vi "Goo00.vi"() -> ()   [LabVIEW 2014]
uses:
  <vilib>/myRIO/Instrument Drivers/Onboard IO/AI/vis/Read.vi
  <vilib>/myRIO/Instrument Drivers/Onboard IO/AI/vis/Smart Open.vi
  <vilib>/Utility/error.llb/Error Cluster From Error Code.vi
  <vilib>/myRIO/Common/Instrument Driver Framework/myRIO v1.0/AI/vis/myRIO v1.0 Read AI.vi
panel:
  out "원소의 인덱스":i32
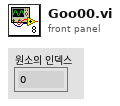
[diagram p1: front panel]
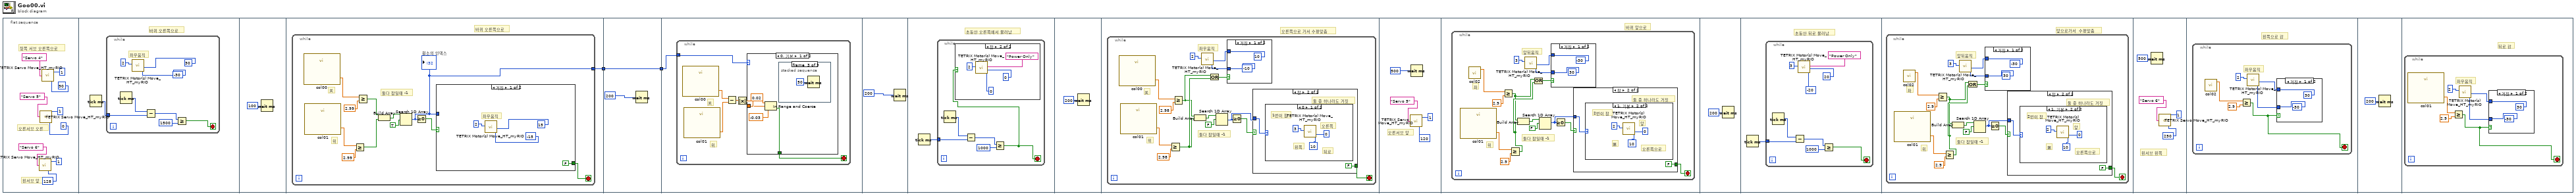
[diagram p0: block diagram]
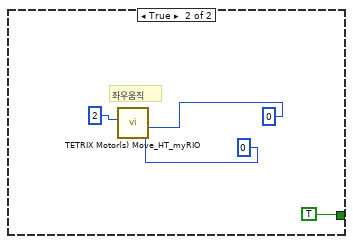
[diagram p2: hidden frame]
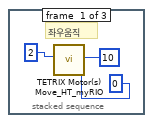
[diagram p3: hidden frame]
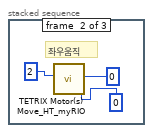
[diagram p4: hidden frame]
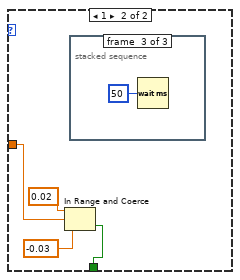
[diagram p5: hidden frame]
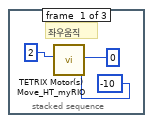
[diagram p6: hidden frame]
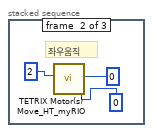
[diagram p7: hidden frame]
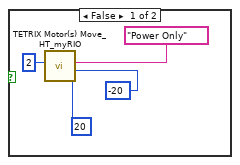
[diagram p8: hidden frame]
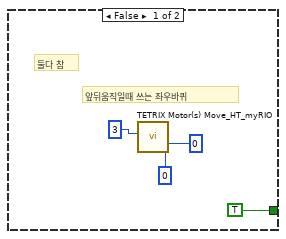
[diagram p9: hidden frame]
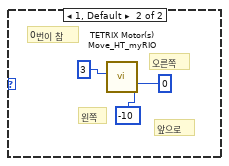
[diagram p10: hidden frame]
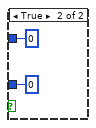
[diagram p11: hidden frame]
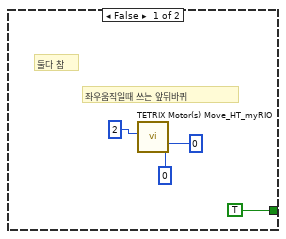
[diagram p12: hidden frame]
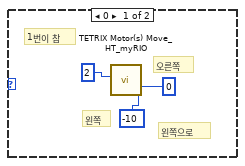
[diagram p13: hidden frame]
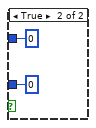
[diagram p14: hidden frame]
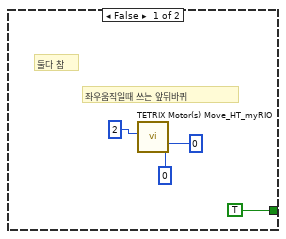
[diagram p15: hidden frame]
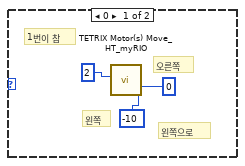
[diagram p16: hidden frame]
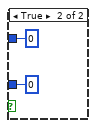
[diagram p17: hidden frame]
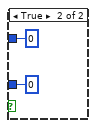
[diagram p18: hidden frame]
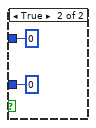
[diagram p19: hidden frame]
diagram:
  n1 = flat-sequence {
    tunnel: [w22] -> w1
    tunnel: [w42] -> w2
    tunnel: w1 -> [w42]
    tunnel: w2 -> [w44]
    frame #0 {
      # "왼서브 앞"
      # "오른서브 오른"
      # "뒷쪽 서브 오른쪽으로"
      n2 = call <vilib>:"TETRIX Servo Move_HT_myRIO.vi"("Servo Position (0 - 255)"=u8 128, "Controller Daisy Chain Position (1 - 4)"=u8 1, "Select Servo"="Servo 6") -> ()  [unwired: 2 in, 1 out]
      n3 = call <vilib>:"TETRIX Servo Move_HT_myRIO.vi"("Servo Position (0 - 255)"=u8 0, "Controller Daisy Chain Position (1 - 4)"=u8 1, "Select Servo"="Servo 5") -> ()  [unwired: 2 in, 1 out]
      n4 = call <vilib>:"TETRIX Servo Move_HT_myRIO.vi"("Servo Position (0 - 255)"=u8 90, "Controller Daisy Chain Position (1 - 4)"=u8 1, "Select Servo"="Servo 4") -> ()  [unwired: 2 in, 1 out]
    }
    frame #1 {
      # "바퀴 오른쪽으로"
      n5 = Tick Count (ms)() -> (millisecond timer value=w12:u32)
      n6 = while {
        tunnel: w12 -> [w16]
        stop <- w13 stop-if-true
        # "좌우움직"
        n7 = Tick Count (ms)() -> (millisecond timer value=w17:u32)
        n8 = call <vilib>:"TETRIX Motor(s) Move_HT_myRIO.vi"("Motor 2 Power (-100 to 100)\n0 = Stop/Brake\n-128 = Stop/Coast"=i8 -30 ("Motor 2 Power (-100 to 100)\n0 = Stop/Brake\n-128 = Stop/Coast"), "Motor 1 Power (-100 to 100)\n0 = Stop/Brake\n-128 = Stop/Coast"=i8 30 ("Motor 1 Power (-100 to 100)\n0 = Stop/Brake\n-128 = Stop/Coast"), "Controller Daisy Chain Position: 1 - 4"=u8 2) -> ()  [unwired: 6 in, 1 out]
        n9 = Subtract(x=w17, y=w16) -> (x-y=w15:u32)
        n10 = Greater Or Equal?(x=w15, y=u32 1500) -> (x >= y?=w13:bool)
      }
    }
    frame #2 {
      n11 = Wait (ms)(milliseconds to wait=u32 100 ("대기 시간(ms)")) -> ()  [unwired: 1 out]
    }
    frame #3 {
      # "바퀴 오른쪽으로"
      n12 = while {
        tunnel: [w23] -> w22
        stop <- w26 stop-if-true
        # "위"
        # "关"
        # "둘다 참일때 -1"
        n13 = call "col00.vi"() -> ("Col00 (B/AI0 (Pin 3))"=w25:dbl)  [unwired: 26 in, 1 out]
        n14 = call "col01.vi"() -> ("Col01 (B/AI1 (Pin 5))"=w24:dbl)  [unwired: 26 in, 1 out]
        n15 = Greater Or Equal?(x=w24, y=2.99) -> (x >= y?=w30:bool)
        n16 = Greater Or Equal?(x=w25, y=2.99) -> (x >= y?=w29:bool)
        n17 = Build Array(w29, w30) -> (w33:bool[])
        n18 = Search 1D Array(1D array=w33, element=TRUE ("원소")) -> (index of element=w23:i32)  [unwired: 1 in]
        "원소의 인덱스" <- w23
        n19 = Greater Or Equal To 0?(x=w23) -> (x >= 0?=w31:bool)
        n20 = case shown="거짓" w31 {
          tunnel: w23 -> [_ _]
          tunnel: [FALSE TRUE] -> w26
          frame False {
            # "좌우움직"
            n21 = call <vilib>:"TETRIX Motor(s) Move_HT_myRIO.vi"("Motor 2 Power (-100 to 100)\n0 = Stop/Brake\n-128 = Stop/Coast"=i8 -15 ("Motor 2 Power (-100 to 100)\n0 = Stop/Brake\n-128 = Stop/Coast"), "Motor 1 Power (-100 to 100)\n0 = Stop/Brake\n-128 = Stop/Coast"=i8 15 ("Motor 1 Power (-100 to 100)\n0 = Stop/Brake\n-128 = Stop/Coast"), "Controller Daisy Chain Position: 1 - 4"=u8 2) -> ()  [unwired: 6 in, 1 out]
          }
          frame True {
            # "좌우움직"
            n22 = call <vilib>:"TETRIX Motor(s) Move_HT_myRIO.vi"("Motor 2 Power (-100 to 100)\n0 = Stop/Brake\n-128 = Stop/Coast"=i8 0 ("Motor 2 Power (-100 to 100)\n0 = Stop/Brake\n-128 = Stop/Coast"), "Motor 1 Power (-100 to 100)\n0 = Stop/Brake\n-128 = Stop/Coast"=i8 0 ("Motor 1 Power (-100 to 100)\n0 = Stop/Brake\n-128 = Stop/Coast"), "Controller Daisy Chain Position: 1 - 4"=u8 2) -> ()  [unwired: 6 in, 1 out]
          }
        }
      }
    }
    frame #4 {
      n23 = Wait (ms)(milliseconds to wait=u32 200 ("대기 시간(ms)")) -> ()  [unwired: 1 out]
    }
    frame #5 {
      n24 = while {
        tunnel: w44 -> [w50]
        stop <- w45 stop-if-true
        # "위"
        # "关"
        n25 = call "col00.vi"() -> ("Col00 (B/AI0 (Pin 3))"=w49:dbl)  [unwired: 26 in, 1 out]
        n26 = call "col01.vi"() -> ("Col01 (B/AI1 (Pin 5))"=w48:dbl)  [unwired: 26 in, 1 out]
        n27 = Subtract(x=w49, y=w48) -> (x-y=w47:dbl)
        n28 = Absolute Value(x=w47) -> (abs(x)=w46:dbl)
        n29 = case shown="0, 기본" w50 {
          tunnel: w46 -> [w54 w63]
          tunnel: [w51 w62] -> w45
          frame 0, Default {
            n30 = In Range and Coerce(upper limit=0.02 ("상위 리미트"), x=w54, lower limit=-0.03 ("상위 리미트")) -> (In Range?=w51:bool)  [unwired: 1 out]
            n31 = stacked-sequence {
              frame #0 {
                # "좌우움직"
                n32 = call <vilib>:"TETRIX Motor(s) Move_HT_myRIO.vi"("Motor 2 Power (-100 to 100)\n0 = Stop/Brake\n-128 = Stop/Coast"=i8 0 ("Motor 2 Power (-100 to 100)\n0 = Stop/Brake\n-128 = Stop/Coast"), "Motor 1 Power (-100 to 100)\n0 = Stop/Brake\n-128 = Stop/Coast"=i8 10 ("Motor 1 Power (-100 to 100)\n0 = Stop/Brake\n-128 = Stop/Coast"), "Controller Daisy Chain Position: 1 - 4"=u8 2) -> ()  [unwired: 6 in, 1 out]
              }
              frame #1 {
                # "좌우움직"
                n33 = call <vilib>:"TETRIX Motor(s) Move_HT_myRIO.vi"("Motor 2 Power (-100 to 100)\n0 = Stop/Brake\n-128 = Stop/Coast"=i8 0 ("Motor 2 Power (-100 to 100)\n0 = Stop/Brake\n-128 = Stop/Coast"), "Motor 1 Power (-100 to 100)\n0 = Stop/Brake\n-128 = Stop/Coast"=i8 0 ("Motor 1 Power (-100 to 100)\n0 = Stop/Brake\n-128 = Stop/Coast"), "Controller Daisy Chain Position: 1 - 4"=u8 2) -> ()  [unwired: 6 in, 1 out]
              }
              frame #2 {
                n34 = Wait (ms)(milliseconds to wait=u32 50 ("대기 시간(ms)")) -> ()  [unwired: 1 out]
              }
            }
          }
          frame 1 {
            n35 = In Range and Coerce(upper limit=0.02 ("상위 리미트"), x=w63, lower limit=-0.03 ("상위 리미트")) -> (In Range?=w62:bool)  [unwired: 1 out]
            n36 = stacked-sequence {
              frame #0 {
                # "좌우움직"
                n37 = call <vilib>:"TETRIX Motor(s) Move_HT_myRIO.vi"("Motor 2 Power (-100 to 100)\n0 = Stop/Brake\n-128 = Stop/Coast"=i8 -10 ("Motor 2 Power (-100 to 100)\n0 = Stop/Brake\n-128 = Stop/Coast"), "Motor 1 Power (-100 to 100)\n0 = Stop/Brake\n-128 = Stop/Coast"=i8 0 ("Motor 1 Power (-100 to 100)\n0 = Stop/Brake\n-128 = Stop/Coast"), "Controller Daisy Chain Position: 1 - 4"=u8 2) -> ()  [unwired: 6 in, 1 out]
              }
              frame #1 {
                # "좌우움직"
                n38 = call <vilib>:"TETRIX Motor(s) Move_HT_myRIO.vi"("Motor 2 Power (-100 to 100)\n0 = Stop/Brake\n-128 = Stop/Coast"=i8 0 ("Motor 2 Power (-100 to 100)\n0 = Stop/Brake\n-128 = Stop/Coast"), "Motor 1 Power (-100 to 100)\n0 = Stop/Brake\n-128 = Stop/Coast"=i8 0 ("Motor 1 Power (-100 to 100)\n0 = Stop/Brake\n-128 = Stop/Coast"), "Controller Daisy Chain Position: 1 - 4"=u8 2) -> ()  [unwired: 6 in, 1 out]
              }
              frame #2 {
                n39 = Wait (ms)(milliseconds to wait=u32 50 ("대기 시간(ms)")) -> ()  [unwired: 1 out]
              }
            }
          }
        }
      }
    }
    frame #6 {
      n40 = Wait (ms)(milliseconds to wait=u32 200 ("대기 시간(ms)")) -> ()  [unwired: 1 out]
    }
    frame #7 {
      # "초동안 오른쪽에서 물러남"
      n41 = Tick Count (ms)() -> (millisecond timer value=w74:u32)
      n42 = while {
        tunnel: w74 -> [w78]
        stop <- w75 stop-if-true
        n43 = Tick Count (ms)() -> (millisecond timer value=w79:u32)
        n44 = Subtract(x=w79, y=w78) -> (x-y=w77:u32)
        n45 = Greater Or Equal?(x=w77, y=u32 1000) -> (x >= y?=w75:bool)
        n46 = case shown="참" w75 {
          frame False {
            n47 = call <vilib>:"TETRIX Motor(s) Move_HT_myRIO.vi"("Motor 2 Power (-100 to 100)\n0 = Stop/Brake\n-128 = Stop/Coast"=i8 20 ("Motor 2 Power (-100 to 100)\n0 = Stop/Brake\n-128 = Stop/Coast"), "Motor 1 Power (-100 to 100)\n0 = Stop/Brake\n-128 = Stop/Coast"=i8 -20 ("Motor 1 Power (-100 to 100)\n0 = Stop/Brake\n-128 = Stop/Coast"), "Control Mode"="Power Only", "Controller Daisy Chain Position: 1 - 4"=u8 2) -> ()  [unwired: 5 in, 1 out]
          }
          frame True {
            n48 = call <vilib>:"TETRIX Motor(s) Move_HT_myRIO.vi"("Motor 2 Power (-100 to 100)\n0 = Stop/Brake\n-128 = Stop/Coast"=i8 0 ("Motor 2 Power (-100 to 100)\n0 = Stop/Brake\n-128 = Stop/Coast"), "Motor 1 Power (-100 to 100)\n0 = Stop/Brake\n-128 = Stop/Coast"=i8 0 ("Motor 1 Power (-100 to 100)\n0 = Stop/Brake\n-128 = Stop/Coast"), "Control Mode"="Power Only", "Controller Daisy Chain Position: 1 - 4"=u8 2) -> ()  [unwired: 5 in, 1 out]
          }
        }
      }
    }
    frame #8 {
      n49 = Wait (ms)(milliseconds to wait=u32 200 ("대기 시간(ms)")) -> ()  [unwired: 1 out]
    }
    frame #9 {
      # "오른쪽으로 가서 수평맞춤"
      n50 = while {
        stop <- w93 stop-if-true
        # "위"
        # "关"
        # "둘다 참일때 -1"
        # "좌우움직"
        n51 = call "col00.vi"() -> ("Col00 (B/AI0 (Pin 3))"=w91:dbl)  [unwired: 26 in, 1 out]
        n52 = call "col01.vi"() -> ("Col01 (B/AI1 (Pin 5))"=w92:dbl)  [unwired: 26 in, 1 out]
        n53 = Greater Or Equal?(x=w92, y=2.98) -> (x >= y?=w95:bool)
        n54 = Greater Or Equal?(x=w91, y=2.98) -> (x >= y?=w94:bool)
        n55 = Build Array(w94, w95) -> (w100:bool[])
        n56 = Or(x=w94, y=w95) -> (x .or. y?=w96:bool)
        n57 = Search 1D Array(1D array=w100, element=FALSE ("원소")) -> (index of element=w97:i32)  [unwired: 1 in]
        n58 = case shown="거짓" w96 {
          tunnel: [i8 10 ("Motor 1 Power (-100 to 100)\n0 = Stop/Brake\n-128 = Stop/Coast") i8 0 ("Motor 1 Power (-100 to 100)\n0 = Stop/Brake\n-128 = Stop/Coast")] -> w102
          tunnel: [i8 -10 ("Motor 2 Power (-100 to 100)\n0 = Stop/Brake\n-128 = Stop/Coast") i8 0 ("Motor 2 Power (-100 to 100)\n0 = Stop/Brake\n-128 = Stop/Coast")] -> w101
          frame False {
          }
          frame True {
          }
        }
        n59 = call <vilib>:"TETRIX Motor(s) Move_HT_myRIO.vi"("Motor 2 Power (-100 to 100)\n0 = Stop/Brake\n-128 = Stop/Coast"=w101, "Motor 1 Power (-100 to 100)\n0 = Stop/Brake\n-128 = Stop/Coast"=w102, "Controller Daisy Chain Position: 1 - 4"=u8 2) -> ()  [unwired: 6 in, 1 out]
        n60 = Greater Or Equal To 0?(x=w97) -> (x >= 0?=w98:bool)
        n61 = case shown="참" w98 {
          tunnel: w97 -> [_ w109]
          tunnel: [TRUE FALSE] -> w93
          frame False {
            # "앞뒤움직일때 쓰는 좌우바퀴"
            # "둘다 참"
            n62 = call <vilib>:"TETRIX Motor(s) Move_HT_myRIO.vi"("Motor 2 Power (-100 to 100)\n0 = Stop/Brake\n-128 = Stop/Coast"=i8 0 ("Motor 2 Power (-100 to 100)\n0 = Stop/Brake\n-128 = Stop/Coast"), "Motor 1 Power (-100 to 100)\n0 = Stop/Brake\n-128 = Stop/Coast"=i8 0 ("Motor 1 Power (-100 to 100)\n0 = Stop/Brake\n-128 = Stop/Coast"), "Controller Daisy Chain Position: 1 - 4"=u8 3) -> ()  [unwired: 6 in, 1 out]
          }
          frame True {
            # "둘 중 하나라도 거짓"
            n63 = case shown="0" w109 {
              frame 0 {
                # "뒤로"
                # "왼쪽"
                # "오른쪽"
                # "1번이 참"
                n64 = call <vilib>:"TETRIX Motor(s) Move_HT_myRIO.vi"("Motor 2 Power (-100 to 100)\n0 = Stop/Brake\n-128 = Stop/Coast"=i8 10 ("Motor 2 Power (-100 to 100)\n0 = Stop/Brake\n-128 = Stop/Coast"), "Motor 1 Power (-100 to 100)\n0 = Stop/Brake\n-128 = Stop/Coast"=i8 0 ("Motor 1 Power (-100 to 100)\n0 = Stop/Brake\n-128 = Stop/Coast"), "Controller Daisy Chain Position: 1 - 4"=u8 3) -> ()  [unwired: 6 in, 1 out]
              }
              frame 1, Default {
                # "앞으로"
                # "왼쪽"
                # "오른쪽"
                # "0번이 참"
                n65 = call <vilib>:"TETRIX Motor(s) Move_HT_myRIO.vi"("Motor 2 Power (-100 to 100)\n0 = Stop/Brake\n-128 = Stop/Coast"=i8 -10 ("Motor 2 Power (-100 to 100)\n0 = Stop/Brake\n-128 = Stop/Coast"), "Motor 1 Power (-100 to 100)\n0 = Stop/Brake\n-128 = Stop/Coast"=i8 0 ("Motor 1 Power (-100 to 100)\n0 = Stop/Brake\n-128 = Stop/Coast"), "Controller Daisy Chain Position: 1 - 4"=u8 3) -> ()  [unwired: 6 in, 1 out]
              }
            }
          }
        }
      }
    }
    frame #10 {
      # "오른서브 앞"
      n66 = call <vilib>:"TETRIX Servo Move_HT_myRIO.vi"("Servo Position (0 - 255)"=u8 120, "Controller Daisy Chain Position (1 - 4)"=u8 1, "Select Servo"="Servo 5") -> ()  [unwired: 2 in, 1 out]
      n67 = Wait (ms)(milliseconds to wait=u32 500 ("대기 시간(ms)")) -> ()  [unwired: 1 out]
    }
    frame #11 {
      # "바퀴 앞으로"
      n68 = while {
        stop <- w132 stop-if-true
        # "위"
        # "둘다 참일때 -1"
        # "앞뒤움직"
        # "좌"
        n69 = call "col01.vi"() -> ("Col01 (B/AI1 (Pin 5))"=w131:dbl)  [unwired: 26 in, 1 out]
        n70 = call "col02.vi"() -> ("Col02 (B/AI2 (Pin 7))"=w128:dbl)  [unwired: 26 in, 1 out]
        n71 = Greater Or Equal?(x=w128, y=2.9) -> (x >= y?=w124:bool)
        n72 = Greater Or Equal?(x=w131, y=2.9) -> (x >= y?=w125:bool)
        n73 = Build Array(w124, w125) -> (w127:bool[])
        n74 = Or(x=w124, y=w125) -> (x .or. y?=w133:bool)
        n75 = Search 1D Array(1D array=w127, element=FALSE ("원소")) -> (index of element=w134:i32)  [unwired: 1 in]
        n76 = case shown="거짓" w133 {
          tunnel: [i8 -30 ("Motor 1 Power (-100 to 100)\n0 = Stop/Brake\n-128 = Stop/Coast") i8 0 ("Motor 1 Power (-100 to 100)\n0 = Stop/Brake\n-128 = Stop/Coast")] -> w137
          tunnel: [i8 30 ("Motor 2 Power (-100 to 100)\n0 = Stop/Brake\n-128 = Stop/Coast") i8 0 ("Motor 2 Power (-100 to 100)\n0 = Stop/Brake\n-128 = Stop/Coast")] -> w136
          frame False {
          }
          frame True {
          }
        }
        n77 = call <vilib>:"TETRIX Motor(s) Move_HT_myRIO.vi"("Motor 2 Power (-100 to 100)\n0 = Stop/Brake\n-128 = Stop/Coast"=w136, "Motor 1 Power (-100 to 100)\n0 = Stop/Brake\n-128 = Stop/Coast"=w137, "Controller Daisy Chain Position: 1 - 4"=u8 3) -> ()  [unwired: 6 in, 1 out]
        n78 = Greater Or Equal To 0?(x=w134) -> (x >= 0?=w135:bool)
        n79 = case shown="참" w135 {
          tunnel: w134 -> [_ w144]
          tunnel: [TRUE FALSE] -> w132
          frame False {
            # "좌우움직일때 쓰는 앞뒤바퀴"
            # "둘다 참"
            n80 = call <vilib>:"TETRIX Motor(s) Move_HT_myRIO.vi"("Motor 2 Power (-100 to 100)\n0 = Stop/Brake\n-128 = Stop/Coast"=i8 0 ("Motor 2 Power (-100 to 100)\n0 = Stop/Brake\n-128 = Stop/Coast"), "Motor 1 Power (-100 to 100)\n0 = Stop/Brake\n-128 = Stop/Coast"=i8 0 ("Motor 1 Power (-100 to 100)\n0 = Stop/Brake\n-128 = Stop/Coast"), "Controller Daisy Chain Position: 1 - 4"=u8 2) -> ()  [unwired: 6 in, 1 out]
          }
          frame True {
            # "둘 중 하나라도 거짓"
            n81 = case shown="1, 기본" w144 {
              frame 0 {
                # "왼쪽으로"
                # "왼쪽"
                # "오른쪽"
                # "1번이 참"
                n82 = call <vilib>:"TETRIX Motor(s) Move_HT_myRIO.vi"("Motor 2 Power (-100 to 100)\n0 = Stop/Brake\n-128 = Stop/Coast"=i8 -10 ("Motor 2 Power (-100 to 100)\n0 = Stop/Brake\n-128 = Stop/Coast"), "Motor 1 Power (-100 to 100)\n0 = Stop/Brake\n-128 = Stop/Coast"=i8 0 ("Motor 1 Power (-100 to 100)\n0 = Stop/Brake\n-128 = Stop/Coast"), "Controller Daisy Chain Position: 1 - 4"=u8 2) -> ()  [unwired: 6 in, 1 out]
              }
              frame 1, Default {
                # "오른쪽으로"
                # "第"
                # "앞"
                # "2번이 참"
                n83 = call <vilib>:"TETRIX Motor(s) Move_HT_myRIO.vi"("Motor 2 Power (-100 to 100)\n0 = Stop/Brake\n-128 = Stop/Coast"=i8 10 ("Motor 2 Power (-100 to 100)\n0 = Stop/Brake\n-128 = Stop/Coast"), "Motor 1 Power (-100 to 100)\n0 = Stop/Brake\n-128 = Stop/Coast"=i8 0 ("Motor 1 Power (-100 to 100)\n0 = Stop/Brake\n-128 = Stop/Coast"), "Controller Daisy Chain Position: 1 - 4"=u8 2) -> ()  [unwired: 6 in, 1 out]
              }
            }
          }
        }
      }
    }
    frame #12 {
      n84 = Wait (ms)(milliseconds to wait=u32 200 ("대기 시간(ms)")) -> ()  [unwired: 1 out]
    }
    frame #13 {
      # "초동안 뒤로 물러남"
      n85 = Tick Count (ms)() -> (millisecond timer value=w156:u32)
      n86 = while {
        tunnel: w156 -> [w162]
        stop <- w159 stop-if-true
        n87 = Tick Count (ms)() -> (millisecond timer value=w163:u32)
        n88 = Subtract(x=w163, y=w162) -> (x-y=w161:u32)
        n89 = call <vilib>:"TETRIX Motor(s) Move_HT_myRIO.vi"("Motor 2 Power (-100 to 100)\n0 = Stop/Brake\n-128 = Stop/Coast"=i8 -20 ("Motor 2 Power (-100 to 100)\n0 = Stop/Brake\n-128 = Stop/Coast"), "Motor 1 Power (-100 to 100)\n0 = Stop/Brake\n-128 = Stop/Coast"=i8 20 ("Motor 1 Power (-100 to 100)\n0 = Stop/Brake\n-128 = Stop/Coast"), "Control Mode"="Power Only", "Controller Daisy Chain Position: 1 - 4"=u8 3) -> ()  [unwired: 5 in, 1 out]
        n90 = Greater Or Equal?(x=w161, y=u32 1000) -> (x >= y?=w159:bool)
      }
    }
    frame #14 {
      # "앞으로가서  수평맞춤"
      n91 = while {
        stop <- w174 stop-if-true
        # "위"
        # "둘다 참일때 -1"
        # "앞뒤움직"
        # "좌"
        n92 = call "col01.vi"() -> ("Col01 (B/AI1 (Pin 5))"=w173:dbl)  [unwired: 26 in, 1 out]
        n93 = call "col02.vi"() -> ("Col02 (B/AI2 (Pin 7))"=w170:dbl)  [unwired: 26 in, 1 out]
        n94 = Greater Or Equal?(x=w170, y=2.9) -> (x >= y?=w166:bool)
        n95 = Greater Or Equal?(x=w173, y=2.9) -> (x >= y?=w167:bool)
        n96 = Build Array(w166, w167) -> (w169:bool[])
        n97 = Or(x=w166, y=w167) -> (x .or. y?=w175:bool)
        n98 = Search 1D Array(1D array=w169, element=FALSE ("원소")) -> (index of element=w176:i32)  [unwired: 1 in]
        n99 = case shown="거짓" w175 {
          tunnel: [i8 -30 ("Motor 1 Power (-100 to 100)\n0 = Stop/Brake\n-128 = Stop/Coast") i8 0 ("Motor 1 Power (-100 to 100)\n0 = Stop/Brake\n-128 = Stop/Coast")] -> w179
          tunnel: [i8 30 ("Motor 2 Power (-100 to 100)\n0 = Stop/Brake\n-128 = Stop/Coast") i8 0 ("Motor 2 Power (-100 to 100)\n0 = Stop/Brake\n-128 = Stop/Coast")] -> w178
          frame False {
          }
          frame True {
          }
        }
        n100 = call <vilib>:"TETRIX Motor(s) Move_HT_myRIO.vi"("Motor 2 Power (-100 to 100)\n0 = Stop/Brake\n-128 = Stop/Coast"=w178, "Motor 1 Power (-100 to 100)\n0 = Stop/Brake\n-128 = Stop/Coast"=w179, "Controller Daisy Chain Position: 1 - 4"=u8 3) -> ()  [unwired: 6 in, 1 out]
        n101 = Greater Or Equal To 0?(x=w176) -> (x >= 0?=w177:bool)
        n102 = case shown="참" w177 {
          tunnel: w176 -> [_ w186]
          tunnel: [TRUE FALSE] -> w174
          frame False {
            # "좌우움직일때 쓰는 앞뒤바퀴"
            # "둘다 참"
            n103 = call <vilib>:"TETRIX Motor(s) Move_HT_myRIO.vi"("Motor 2 Power (-100 to 100)\n0 = Stop/Brake\n-128 = Stop/Coast"=i8 0 ("Motor 2 Power (-100 to 100)\n0 = Stop/Brake\n-128 = Stop/Coast"), "Motor 1 Power (-100 to 100)\n0 = Stop/Brake\n-128 = Stop/Coast"=i8 0 ("Motor 1 Power (-100 to 100)\n0 = Stop/Brake\n-128 = Stop/Coast"), "Controller Daisy Chain Position: 1 - 4"=u8 2) -> ()  [unwired: 6 in, 1 out]
          }
          frame True {
            # "둘 중 하나라도 거짓"
            n104 = case shown="1, 기본" w186 {
              frame 0 {
                # "왼쪽으로"
                # "왼쪽"
                # "오른쪽"
                # "1번이 참"
                n105 = call <vilib>:"TETRIX Motor(s) Move_HT_myRIO.vi"("Motor 2 Power (-100 to 100)\n0 = Stop/Brake\n-128 = Stop/Coast"=i8 -10 ("Motor 2 Power (-100 to 100)\n0 = Stop/Brake\n-128 = Stop/Coast"), "Motor 1 Power (-100 to 100)\n0 = Stop/Brake\n-128 = Stop/Coast"=i8 0 ("Motor 1 Power (-100 to 100)\n0 = Stop/Brake\n-128 = Stop/Coast"), "Controller Daisy Chain Position: 1 - 4"=u8 2) -> ()  [unwired: 6 in, 1 out]
              }
              frame 1, Default {
                # "오른쪽으로"
                # "第"
                # "앞"
                # "2번이 참"
                n106 = call <vilib>:"TETRIX Motor(s) Move_HT_myRIO.vi"("Motor 2 Power (-100 to 100)\n0 = Stop/Brake\n-128 = Stop/Coast"=i8 10 ("Motor 2 Power (-100 to 100)\n0 = Stop/Brake\n-128 = Stop/Coast"), "Motor 1 Power (-100 to 100)\n0 = Stop/Brake\n-128 = Stop/Coast"=i8 0 ("Motor 1 Power (-100 to 100)\n0 = Stop/Brake\n-128 = Stop/Coast"), "Controller Daisy Chain Position: 1 - 4"=u8 2) -> ()  [unwired: 6 in, 1 out]
              }
            }
          }
        }
      }
    }
    frame #15 {
      # "왼서브 왼쪽"
      n107 = Wait (ms)(milliseconds to wait=u32 500 ("대기 시간(ms)")) -> ()  [unwired: 1 out]
      n108 = call <vilib>:"TETRIX Servo Move_HT_myRIO.vi"("Servo Position (0 - 255)"=u8 250, "Controller Daisy Chain Position (1 - 4)"=u8 1, "Select Servo"="Servo 6") -> ()  [unwired: 2 in, 1 out]
    }
    frame #16 {
      # "왼쪽으로 감"
      n109 = while {
        stop <- w202 stop-if-true
        # "좌우움직"
        n110 = call "col02.vi"() -> ("Col02 (B/AI2 (Pin 7))"=w201:dbl)  [unwired: 26 in, 1 out]
        n111 = Greater Or Equal?(x=w201, y=2.9) -> (x >= y?=w202:bool)
        n112 = case shown="거짓" w202 {
          tunnel: [i8 30 ("Motor 1 Power (-100 to 100)\n0 = Stop/Brake\n-128 = Stop/Coast") i8 0 ("Motor 1 Power (-100 to 100)\n0 = Stop/Brake\n-128 = Stop/Coast")] -> w204
          tunnel: [i8 -30 ("Motor 2 Power (-100 to 100)\n0 = Stop/Brake\n-128 = Stop/Coast") i8 0 ("Motor 2 Power (-100 to 100)\n0 = Stop/Brake\n-128 = Stop/Coast")] -> w203
          frame False {
          }
          frame True {
          }
        }
        n113 = call <vilib>:"TETRIX Motor(s) Move_HT_myRIO.vi"("Motor 2 Power (-100 to 100)\n0 = Stop/Brake\n-128 = Stop/Coast"=w203, "Motor 1 Power (-100 to 100)\n0 = Stop/Brake\n-128 = Stop/Coast"=w204, "Controller Daisy Chain Position: 1 - 4"=u8 2) -> ()  [unwired: 6 in, 1 out]
      }
    }
    frame #17 {
      n114 = Wait (ms)(milliseconds to wait=u32 200 ("대기 시간(ms)")) -> ()  [unwired: 1 out]
    }
    frame #18 {
      # "뒤로 감"
      n115 = while {
        stop <- w213 stop-if-true
        # "좌우움직"
        n116 = call "col01.vi"() -> ("Col01 (B/AI1 (Pin 5))"=w212:dbl)  [unwired: 26 in, 1 out]
        n117 = Greater Or Equal?(x=w212, y=2.9) -> (x >= y?=w213:bool)
        n118 = case shown="거짓" w213 {
          tunnel: [i8 30 ("Motor 1 Power (-100 to 100)\n0 = Stop/Brake\n-128 = Stop/Coast") i8 0 ("Motor 1 Power (-100 to 100)\n0 = Stop/Brake\n-128 = Stop/Coast")] -> w215
          tunnel: [i8 -30 ("Motor 2 Power (-100 to 100)\n0 = Stop/Brake\n-128 = Stop/Coast") i8 0 ("Motor 2 Power (-100 to 100)\n0 = Stop/Brake\n-128 = Stop/Coast")] -> w214
          frame False {
          }
          frame True {
          }
        }
        n119 = call <vilib>:"TETRIX Motor(s) Move_HT_myRIO.vi"("Motor 2 Power (-100 to 100)\n0 = Stop/Brake\n-128 = Stop/Coast"=w214, "Motor 1 Power (-100 to 100)\n0 = Stop/Brake\n-128 = Stop/Coast"=w215, "Controller Daisy Chain Position: 1 - 4"=u8 2) -> ()  [unwired: 6 in, 1 out]
      }
    }
  }
